vi "clientG3.vi"() -> ()   [LabVIEW 2020]
panel:
  in  "stop":bool
  out "Waveform Chart":dbl(graph)
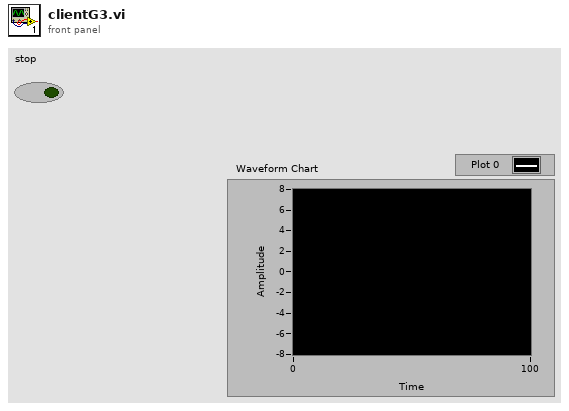
[diagram p1: front panel]
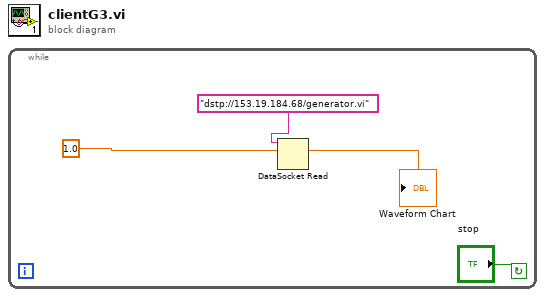
[diagram p0: block diagram]
diagram:
  n1 = while {
    stop <- "stop" continue-if-true
    n2 = DataSocket Read(10:1.0, 11:"dstp://153.19.184.68/generator.vi" ("connection in")) -> (2:→"Waveform Chart":dbl)  [unwired: 3 in, 6 out]
  }
